vi "Parallel Test.vi"(9 "Test Complete Event":refnum<user-event>, 10 "Positions":u32[](array[numeric]), 11 "Parallel Test in":refnum<class "Parallel Test.lvclass">) -> ()   [LabVIEW 2015, in "Parallel Test.lvclass"]
uses:
  Parallel Test.lvclass
  typedefs/Parallel Return -- Cluster.ctl
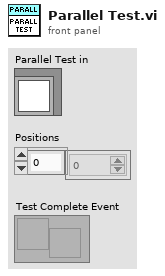
[diagram p1: front panel]
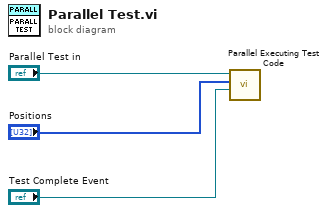
[diagram p0: block diagram]
diagram:
  n1 = call-dynamic "Parallel Executing Test Code.vi"("Test Complete Event"="Test Complete Event", "Positions"="Positions", "Parallel Test in"="Parallel Test in") -> ()  [unwired: 9 in]
